vi "CheckAnalysisSettingValid.vi"(7 "Analysis_Type":T1=enum."G_PatternMatching", 8 "error in (no error)":errorcluster, 11 "ParameterIn":string) -> (0 "error out":errorcluster, 3 "ParameterOut":string, 4 "Valid":bool)   [LabVIEW 2019]
uses:
  Controls/V_Analysis_Type.ctl
  Controls/Analysis_Setting.ctl
  f899d9e6-637b-4d12-bb15-0bfc593db446.vi
  <vilib>/JDP Science/JSONtext/JSON text to Variant.vi
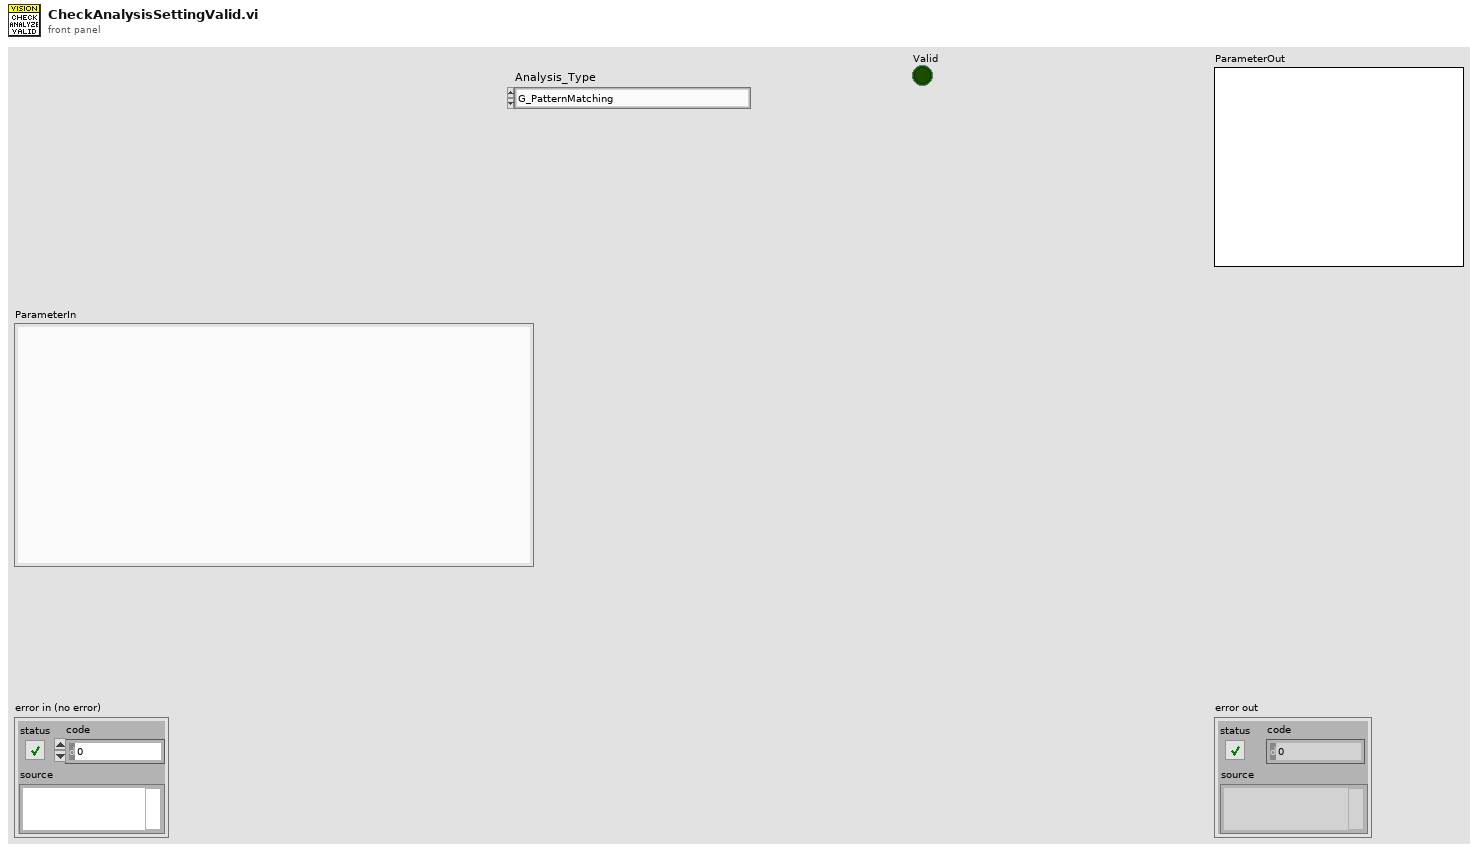
[diagram p1: front panel]
types:
  T1 = typedef "V_Analysis_Type.ctl" = enum16{"None", "C_Color Pattern Matching", "G_PatternMatching", "G_ShapeDectect", "G_GeometricMatch", "B_Area Check"}
  T2 = typedef "Analysis_Setting.ctl" = cluster{"PreProcess":T1, "Parameter":string}
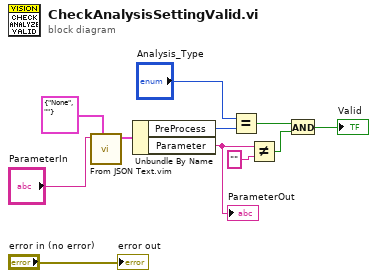
[diagram p0: block diagram]
diagram:
  n1 = call "From JSON Text.vim"("Data Type and Default Value"=T2 {"PreProcess"=enum."None", "Parameter"=""} ("Analysis_Setting In"), "JSON"="ParameterIn") -> ("Data out"=w4:T2)  [unwired: 8 in, 1 out]
  n2 = Unbundle By Name(w4) -> ("PreProcess"=w3:T1, "Parameter"=w2:string)
  "ParameterOut" <- w2
  n3 = Equal?(x="Analysis_Type", y=w3) -> (x = y?=w9:bool)
  n4 = Not Equal?(x=w2, y="") -> (x != y?=w10:bool)
  n5 = And(x=w9, y=w10) -> (x .and. y?=→"Valid":bool)
  "error out" <- "error in (no error)"
